vi "CamServer global.vi"() -> ()   [LabVIEW 2015]
uses:
  Camera enum/Camera enum.ctl
panel:
  in  "Demanded cameras":T1[](array[typedef])=["Travcam", "Tunnelcam", "Pencilcam"]
  in  "CamServer machine name or IP":string="EnFlo-CamServer"
  in  "Scratch file directory":path=path "\\\\EnFlo-Data\\Public/CamServer"
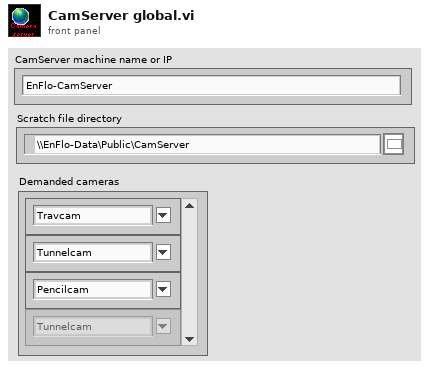
[diagram p1: front panel]
types:
  T1 = typedef "Camera enum.ctl" = string
diagram:
